vi "Actions.vi"(8 "error in (no error)":errorcluster, 11 "CONTROLLER in":refnum<class "CONTROLLER.lvclass">) -> (0 "error out":errorcluster, 3 "CONTROLLER out":refnum<class "CONTROLLER.lvclass">)   [LabVIEW 2013, in "CONTROLLER.lvclass"]
uses:
  CONTROLLER.lvclass
  View/base/VIEW.lvclass
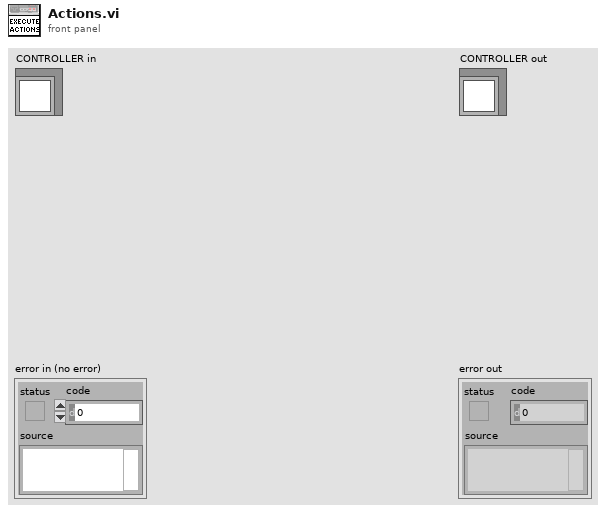
[diagram p1: front panel]
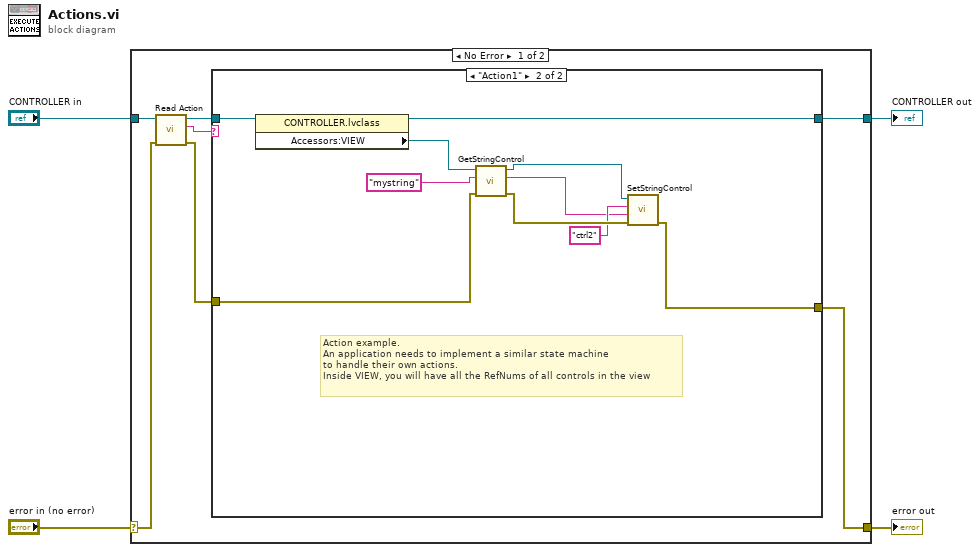
[diagram p0: block diagram]
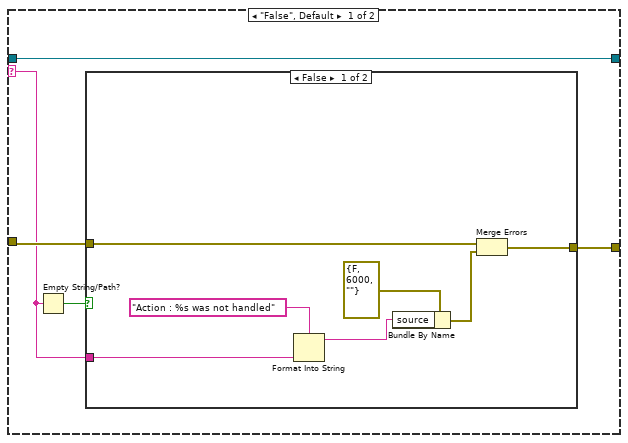
[diagram p2: hidden frame]
diagram:
  n1 = case shown="No Error" "error in (no error)" {
    selector: "error in (no error)" -> [w10 w36]
    tunnel: [w5 w36] -> w3
    tunnel: [w7 w35] -> w1
    tunnel: "CONTROLLER in" -> [w11 w35]
    frame No Error {
      n2 = call-dynamic "Read Action.vi"("error in (no error)"=w10, "CONTROLLER in"=w11) -> ("error out"=w6:errorcluster, "Action"=w9:string, "CONTROLLER out"=w8:refnum<class "CONTROLLER.lvclass">)  [unwired: 7 in]
      n3 = case shown="\"Action1\"" w9 {
        selector: w9 -> [w13 _]
        tunnel: w8 -> [w14 w28]
        tunnel: [w14 w27] -> w7
        tunnel: w6 -> [w15 w26]
        tunnel: [w16 w25] -> w5
        frame "False", Default {
          n4 = Empty String/Path?(string/path=w13) -> (empty?=w12:bool)
          n5 = case shown="False" w12 {
            tunnel: [w21 w24] -> w16
            tunnel: w15 -> [w19 w24]
            tunnel: w13 -> [w17 _]
            frame False {
              n6 = Format Into String(format string="Action : %s was not handled", w17) -> (resulting string=w22:string)  [unwired: 2 in, 1 out]
              n7 = Bundle By Name(cluster=errorcluster {"status"=FALSE, "code"=6000, "source"=""} ("error out"), "source"=w22) -> (w20:errorcluster)
              n8 = Merge Errors(w19, w20) -> (w21:errorcluster)
            }
            frame True {
            }
          }
        }
        frame "Action1" {
          # "Action example.\nAn application needs to implement a similar state machine\nto handle their own actions.\nInside VIEW, you will have all the RefNums of all controls in the view"
          n9 = property class="CONTROLLER.lvclass"(reference=w28) -> (reference out=w27:refnum<class "CONTROLLER.lvclass">, "Accessors:VIEW"=w29:refnum<class "VIEW.lvclass">)  [unwired: 1 in, 1 out]
          n10 = call "GetStringControl.vi"("error in (no error)"=w26, "Name"="mystring", "VIEW in"=w29) -> ("error out"=w34:errorcluster, "Text.Text"=w30:string, "VIEW out"=w32:refnum<class "VIEW.lvclass">)  [unwired: 6 in]
          n11 = call "SetStringControl.vi"("error in (no error)"=w34, "Text.Text"=w30, "Name"="ctrl2", "VIEW in"=w32) -> ("error out"=w25:errorcluster)  [unwired: 6 in, 1 out]
        }
      }
    }
    frame Error {
    }
  }
  "error out" <- w3
  "CONTROLLER out" <- w1
